vi "Get Minor Frame by Name.vi"(8 "error in":errorcluster, 10 "name":string, 11 "BusController in":refnum<k24>) -> (0 "error out":errorcluster, 1 "Minor Frame ref":refnum<k24>, 2 "found":bool, 3 "BusController out":refnum<k24>)   [LabVIEW 2020, in "Ballard_1553_Hardware_ni.lvlib"]
uses:
  Ballard_1553_Hardware_ni.lvlib
  C:/Users/Administrator/Desktop/GIT/Ballard-MIL-STD-1553-Custom-Device/Source/System Explorer/SubVIs/Parse XML Ballard/1.2/BTIXML_SerDes.dll
  Ballard-MIL-STD-1553-Custom-Device/Source/System Explorer/SubVIs/Parse XML Ballard/1.2/BTIXML_SerDes.dll
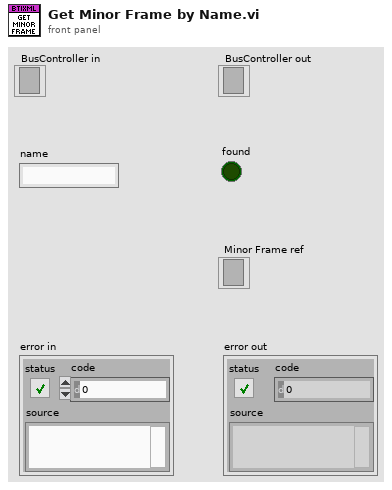
[diagram p1: front panel]
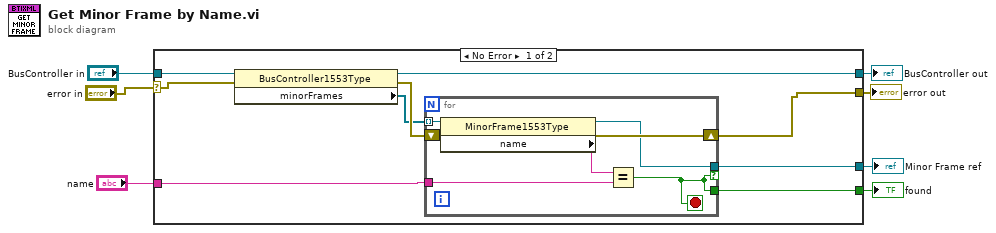
[diagram p0: block diagram]
diagram:
  n1 = case shown="No Error" "error in" {
    selector: "error in" -> [w14 w24]
    tunnel: [w10 w24] -> w7
    tunnel: [w15 w25] -> w6
    tunnel: "BusController in" -> [w16 w25]
    tunnel: "name" -> [w12 _]
    tunnel: [w9 _] -> w2
    tunnel: [w8 _] -> w1
    frame No Error {
      n2 = property class="BusController1553Type"(reference=w16, error in=w14) -> (reference out=w15:refnum<k24>, error out=w13:errorcluster, "minorFrames"=w11:refnum<k24>[])
      n3 = for {
        shift-right: [w19] -> w10
        shift-left: w13 -> [w22]
        tunnel: w12 -> [w20]
        tunnel: w11 -> [w23] mode=indexing
        tunnel: [w18] -> w8 if=w17
        tunnel: [w17] -> w9
        stop <- w17 stop-if-true
        n4 = property class="MinorFrame1553Type"(reference=w23, error in=w22) -> (reference out=w18:refnum<k24>, error out=w19:errorcluster, "name"=w21:string)
        n5 = Equal?(x=w21, y=w20) -> (x = y?=w17:bool)
      }
    }
    frame Error {
    }
  }
  "error out" <- w7
  "BusController out" <- w6
  "found" <- w2
  "Minor Frame ref" <- w1
